vi "ReplaceTemplate PNGs.vi"(6 "Control Destination":path, 8 "error in":errorcluster, 9 "States PNGs":path[](array[path]), 10 "CTL template":path, 11 "Control in":refnum<class "Control.lvclass">) -> (0 "error out":errorcluster, 2 "Control Destination dup":path, 3 "Control out":refnum<class "Control.lvclass">)   [LabVIEW 2012, in "Control.lvclass"]
doc: "Replaces the template button image with the one created from the object's properties."
uses:
  Control.lvclass
  _ResourceManager_v86/ResManager/IDCloneResMgr.lvlib
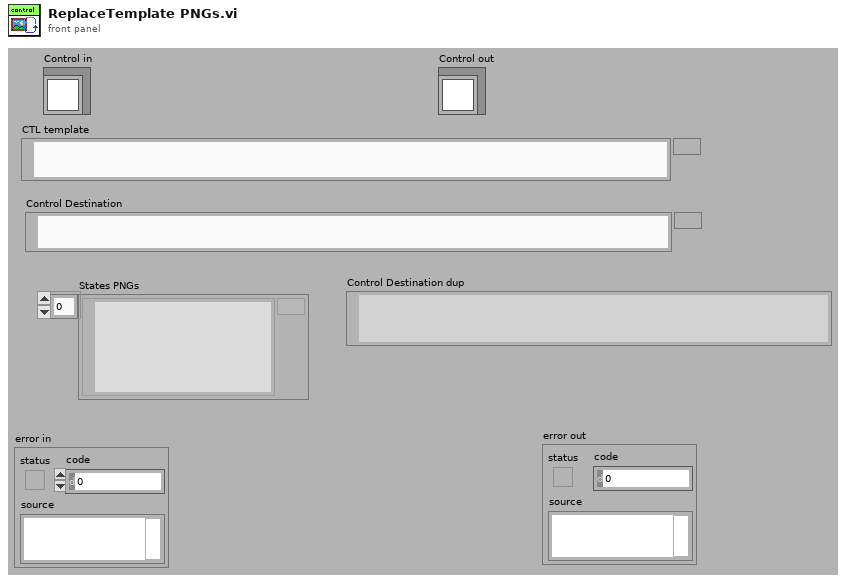
[diagram p1: front panel]
types:
  T1 = typedef "IDCloneResMgr.lvlib/ID_Resource info.ctl" = cluster{"type":u32, "id":i32, "name":string, "binary data":string}
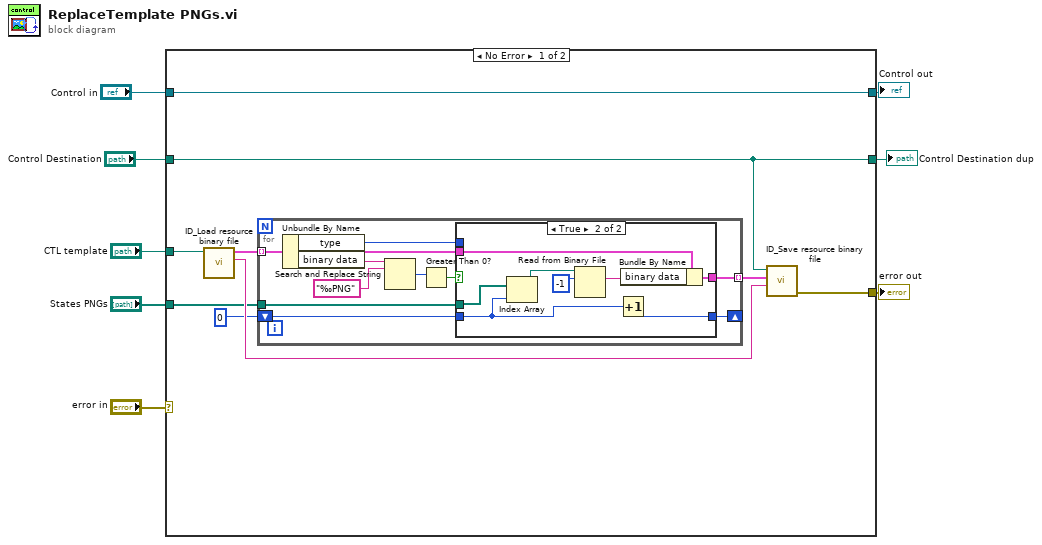
[diagram p0: block diagram]
diagram:
  n1 = case shown="No Error" "error in" {
    selector: "error in" -> [_ w40]
    tunnel: "CTL template" -> [w14 _]
    tunnel: "States PNGs" -> [w13 _]
    tunnel: "Control Destination" -> [w9 w38]
    tunnel: [w11 w40] -> w5
    tunnel: "Control in" -> [w10 w39]
    tunnel: [w10 w39] -> w2
    tunnel: [w9 w38] -> w1
    frame No Error {
      n2 = call "ID_Load resource binary file.vi"("resource binary file"=w14) -> ("file type"=w17:string, "resources"=w15:T1[])  [unwired: 9 out]
      n3 = for {
        tunnel: w15 -> [w19] mode=indexing
        tunnel: [w24] -> w16 mode=indexing
        tunnel: w13 -> [w22]
        shift-right: [w20] -> _
        shift-left: 0 -> [w21]
        n4 = Unbundle By Name(w19) -> ("type"=w18:u32, "binary data"=w27:string)
        n5 = Search and Replace String(input string=w27, search string="‰PNG") -> (number of replacements=w26:i32)  [unwired: 1 in, 8 out]
        n6 = Greater Than 0?(x=w26) -> (x > 0?=w25:bool)
        n7 = case shown="True" w25 {
          tunnel: w19 -> [w29 w37]
          tunnel: [w29 w36] -> w24
          tunnel: w22 -> [_ w33]
          tunnel: w21 -> [w28 w31]
          tunnel: [w28 w30] -> w20
          tunnel: w18 -> [_ _]
          frame False {
          }
          frame True {
            n8 = Index Array(array=w33, index=w31) -> (element=w32:path)
            n9 = Read from Binary File(10:-1 ("count"), 11:w32) -> (2:w34:string)  [unwired: 1 in, 6 out]
            n10 = Increment(x=w31) -> (x+1=w30:i32)
            n11 = Bundle By Name(cluster=w37, "binary data"=w34) -> (w36:T1)
          }
        }
      }
      n12 = call "ID_Save resource binary file.vi"("file type"=w17, "resources"=w16, "resource binary file"=w9) -> ("error out"=w11:errorcluster)  [unwired: 8 out]
    }
    frame Error {
    }
  }
  "error out" <- w5
  "Control out" <- w2
  "Control Destination dup" <- w1
